vi "read default menu name.vi"(8 "error in":errorcluster, 11 "TBM Configuration Node in":refnum<class "TBM Configuration Node.lvclass">) -> (0 "error out":errorcluster, 2 "default menu name":string, 3 "TBM Configuration Node out":refnum<class "TBM Configuration Node.lvclass">)   [LabVIEW 2013, in "PL Framework Configuration Tool.lvlib" / "TBM Configuration Node.lvclass"]
uses:
  TBM Configuration Node.lvclass
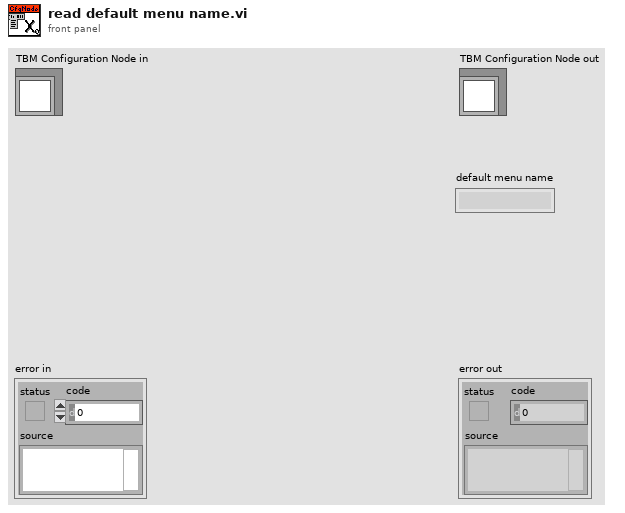
[diagram p1: front panel]
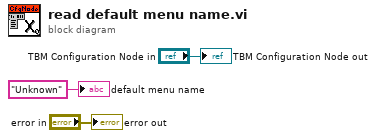
[diagram p0: block diagram]
diagram:
  "error out" <- "error in"
  "TBM Configuration Node out" <- "TBM Configuration Node in"
  "default menu name" <- "Unknown" ("default menu name")
